vi "Open.vi"(8 "error in (no error)":errorcluster, 11 "HAL.Serial in":refnum<class "HAL.Serial.lvclass">) -> (0 "error out":errorcluster, 3 "HAL.Serial out":refnum<class "HAL.Serial.lvclass">)   [LabVIEW 2019, in "Instrument.lvlib" / "HAL.Serial.lvclass"]
uses:
  HAL.Serial.lvclass
  HAL.Serial.lvclass/HAL.Serial.ctl
  <vilib>/Instr/_visa.llb/VISA Configure Serial Port (Instr).vi
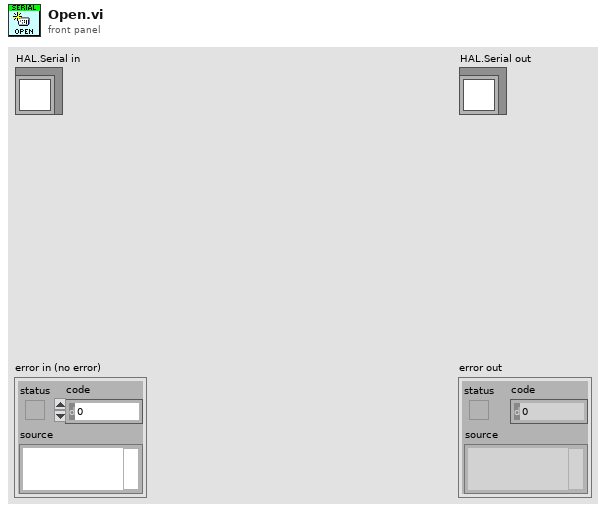
[diagram p1: front panel]
types:
  T1 = typedef "Serial - ASCII Characters.ctl" = enum16{"NUL", "SOH", "STX", "ETX", "EOT", "ENQ", "ACK", "BEL", "BS", "HT", "LF", "VT", "FF", "CR", "SO", "SI", "DLE", "DC1", "DC2", "DC3", "DC4", "NAK", "SYN", "ETB", "CAN", "EM", "SUB", "ESC", "FS", "GS", "RS", "US", "SP", "!", "\"", "#", "$", "%", "&", "'", "(", ")", "*", "+", ",", "- (-)", ".", "/", "0", "1", "2", "3", "4", "5", "6", "7", "8", "9", ":", ";", "<", "=", ">", "?", "@", "A", "B", "C", "D", "E", "F", "G", "H", "I", "J", "K", "L", "M", "N", "O", "P", "Q", "R", "S", "T", "U", "V", "W", "X", "Y", "Z", "[", "\\", "]", "^", "_", "`", "a", "b", "c", "d", "e", "f", "g", "h", "i", "j", "k", "l", "m", "n", "o", "p", "q", "r", "s", "t", "u", "v", "w", "x", "y", "z", "{", "|", "}", "~"}
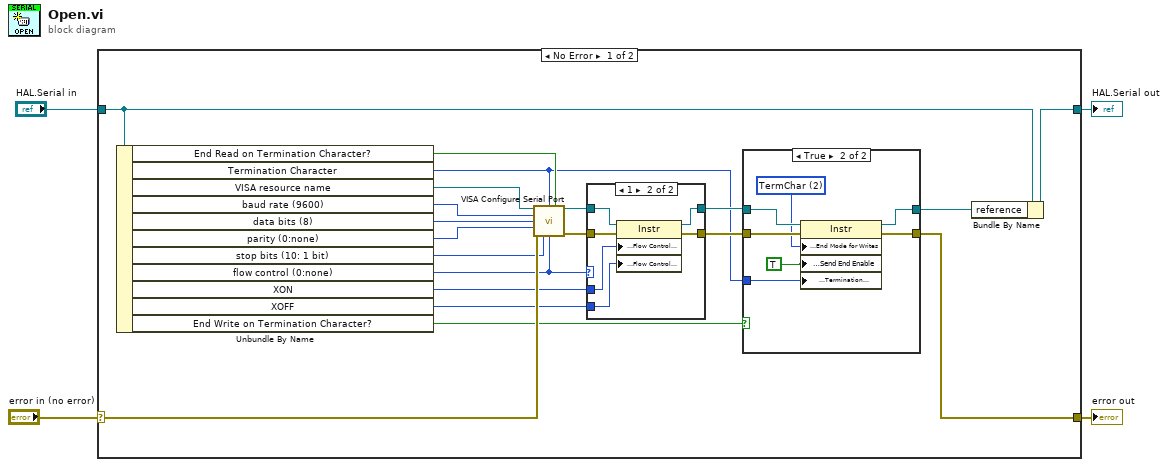
[diagram p0: block diagram]
diagram:
  n1 = case shown="No Error" "error in (no error)" {
    selector: "error in (no error)" -> [w24 w43]
    tunnel: [w7 w43] -> w4
    tunnel: "HAL.Serial in" -> [w22 w42]
    tunnel: [w21 w42] -> w1
    frame No Error {
      n2 = Unbundle By Name(w22) -> ("End Read on Termination Character?"=w23:bool, "Termination Character"=w8:u8, "VISA resource name"=w20:refnum<visa-resource-name>, "baud rate (9600)"=w5:u32, "data bits (8)"=w19:u16, "parity (0:none)"=w6:enum16{"None", "Odd", "Even", "Mark", "Space"}, "stop bits (10: 1 bit)"=w18:u16, "flow control (0:none)"=w17:u16, "XON"=w11:T1, "XOFF"=w10:T1, "End Write on Termination Character?"=w9:bool)
      n3 = call-poly "VISA Configure Serial Port"("VISA resource name"=w20, "termination char\n(0xA = '\\n' = LF)"=w8, "Enable Termination\nChar (T)"=w23, "baud rate (9600)"=w5, "data bits (8)"=w19, "parity (0:none)"=w6, "error in (no error)"=w24, "stop bits (10: 1 bit)"=w18, "flow control (0:none)"=w17) -> ("VISA resource name out"=w16:refnum<visa-resource-name>, "error out"=w15:errorcluster)  [unwired: 5 in]
      n4 = case shown="1" w17 {
        tunnel: [w34 w41] -> w14
        tunnel: [w35 w40] -> w13
        tunnel: w15 -> [w34 w39]
        tunnel: w16 -> [w35 w38]
        tunnel: w11 -> [_ w37]
        tunnel: w10 -> [_ w36]
        frame Default {
        }
        frame 1 {
          n5 = property class="Instr"(reference=w38, error in=w39, "Serial Settings:Flow Control XON Character"=w37, "Serial Settings:Flow Control XOFF Character"=w36) -> (reference out=w40:refnum<visa-resource-name>, error out=w41:errorcluster)
        }
      }
      n6 = case shown="True" w9 {
        tunnel: w13 -> [w25 w33]
        tunnel: w14 -> [w26 w32]
        tunnel: [w25 w31] -> w12
        tunnel: [w26 w30] -> w7
        tunnel: w8 -> [_ w29]
        frame False {
        }
        frame True {
          w27 = u16 2 items=["None", "LastBit", "TermChar", "Break"] ("Serial Settings:Serial End Mode for Writes")
          n7 = property class="Instr"(reference=w33, error in=w32, "Serial Settings:End Mode for Writes"=w27, "Message Based Settings:Send End Enable"=TRUE, "Message Based Settings:Termination Character"=w29) -> (reference out=w31:refnum<visa-resource-name>, error out=w30:errorcluster)
        }
      }
      n8 = Bundle By Name(cluster=w22, "reference"=w12) -> (w21:refnum<class "HAL.Serial.lvclass">)
    }
    frame Error {
    }
  }
  "error out" <- w4
  "HAL.Serial out" <- w1
